vi "Translation3d_GetNorm.vi"(11 "In Translation3d":T1 {"Z" format="%14.3f"; "Y" format="%14.3f"; "X" format="%14.3f"}) -> (3 "Norm":dbl)   [LabVIEW 2019, in "Trajectory_Library.lvlib"]
doc: "Returns the norm, or distance from the origin to the translation.\n\nParameters:\n - IN TRANSLATION - This translation data structure\n\nReturns:\n - Norm - The norm of the translation."
uses:
  Trajectory_Library.lvlib
  TRANSLATION3D.ctl
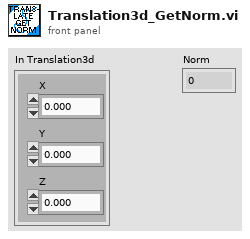
[diagram p1: front panel]
types:
  T1 = typedef "Trajectory_Library.lvlib/TRANSLATION3D.ctl" = cluster{"X":dbl, "Y":dbl, "Z":dbl}
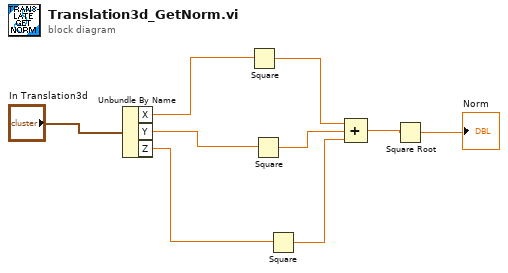
[diagram p0: block diagram]
diagram:
  n1 = Unbundle By Name("In Translation3d") -> ("X"=w4:dbl, "Y"=w3:dbl, "Z"=w2:dbl)
  n2 = Square(x=w4) -> (x^2=w9:dbl)
  n3 = Square(x=w3) -> (x^2=w8:dbl)
  n4 = Square(x=w2) -> (x^2=w7:dbl)
  n5 = Compound Arithmetic op=ADD(w9, w8, w7) -> (w6:dbl)
  n6 = Square Root(x=w6) -> (sqrt(x)=→"Norm":dbl)
